vi "Post-Project-Copying Process - Error Handling.vi"(8 "error in":errorcluster, 11 "PluginGenerator_MetaDataObj":refnum<class "PluginGenerator_MetaDataObj.lvclass">) -> (0 "error out":errorcluster, 3 "PluginGenerator_MetaDataObj out":refnum<class "PluginGenerator_MetaDataObj.lvclass">)   [LabVIEW 2023, in "Plugin Generator.lvlib"]
uses:
  Plugin Generator.lvlib
  PluginGenerator_MetaDataObj/PluginGenerator_MetaDataObj.lvclass
  c:/perforce/build/exports/ni/nito/nitoolchainlabview2023eng64/official/export/23.3/23.3.0f52/win/resource/dialog/NewProjectWizard/MetaDataObj/MetaDataObj.lvclass
  <vilib>/Utility/error.llb/DialogType.ctl
  <resource>/dialog/NewProjectWizard/MetaDataObj/MetaDataObj.lvclass/MetaDataObj.ctl
  <resource>/dialog/NewProjectWizard/MetaDataObj/Accessors/Read Project Root.vi
  <resource>/dialog/NewProjectWizard/MetaDataObj/Accessors/Read Project Name.vi
  <vilib>/dlg_ctls.llb/Space Constant.vi
  [Global].vi
  <resource>/dialog/NewProjectWizard/MetaDataObj/Accessors/Read Project Path.vi
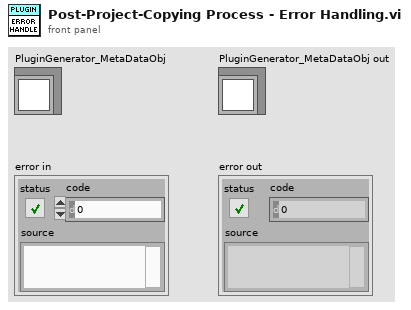
[diagram p1: front panel]
types:
  T1 = typedef "DialogType.ctl" = u16
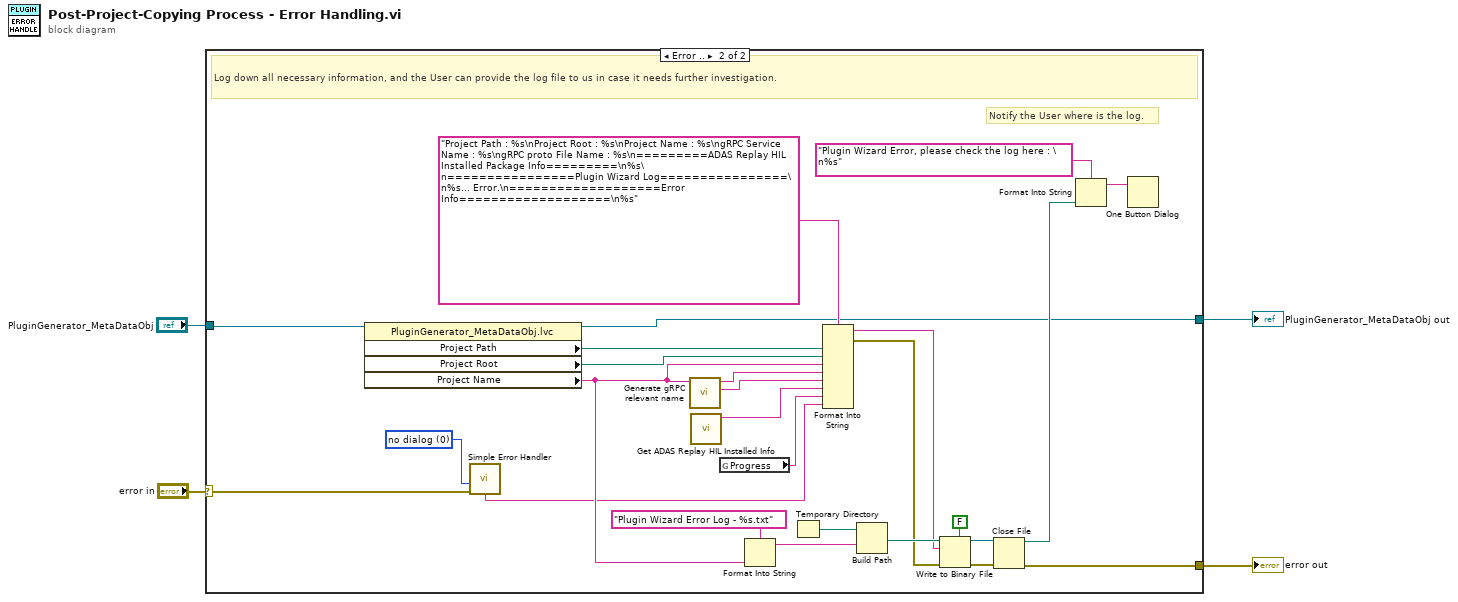
[diagram p0: block diagram]
diagram:
  n1 = case shown="Error .." "error in" {
    selector: "error in" -> [w6 w32]
    tunnel: [w6 w12] -> w4
    tunnel: "PluginGenerator_MetaDataObj" -> [w5 w30]
    tunnel: [w5 w11] -> w1
    frame No Error {
    }
    frame Error {
      w31 = T1 0 items=["no dialog", "OK message", "continue or stop message", "OK message + warnings", "continue/stop + warnings"] ("type of dialog (OK msg:1)")
      # "Notify the User where is the log."
      # "Log down all necessary information, and the User can provide the log file to us in case it needs further investigation."
      n2 = property class="PluginGenerator_MetaDataObj.lvc"(reference=w30) -> (reference out=w11:refnum<class "PluginGenerator_MetaDataObj.lvclass">, "Project Path"=w29:path, "Project Root"=w28:path, "Project Name"=w23:string)  [unwired: 1 in, 1 out]
      n3 = call <vilib>:"Simple Error Handler.vi"("type of dialog (OK msg:1)"=w31, "error in (no error)"=w32) -> ("message"=w9:string)  [unwired: 3 in, 4 out]
      n4 = call "Generate gRPC relevant name.vi"("Project Name"=w23) -> ("gRPC proto File Name"=w26:string, "gRPC Service Name"=w27:string)  [unwired: 9 in]
      n5 = call "Get ADAS Replay HIL Installed Info.vi"() -> ("ADAS Replay HIL pkg info"=w7:string)  [unwired: 11 in]
      n6 = global read "[Global].vi" "Progress"() -> (w8:string)
      n7 = Format Into String(format string="Plugin Wizard Error Log - %s.txt", w23) -> (resulting string=w21:string)  [unwired: 2 in, 1 out]
      n8 = Temporary Directory() -> (w24:path)
      n9 = Format Into String(format string="Project Path : %s\nProject Root : %s\nProject Name : %s\ngRPC Service Name : %s\ngRPC proto File Name : %s\n=========ADAS Replay HIL Installed Package Info=========\n%s\n================Plugin Wizard Log================\n%s... Error.\n===================Error Info===================\n%s", w29, w28, w23, w27, w26, w7, w8, w9) -> (resulting string=w19:string, error out=w18:errorcluster)  [unwired: 2 in]
      n10 = Build Path(base path=w24, name or relative path=w21) -> (appended path=w20:path)
      n11 = Write to Binary File(file (use dialog)=w20, data=w19, error in=w18, 5:FALSE ("prepend array or string size? (T)")) -> (refnum out=w16:refnum<file>, error out=w17:errorcluster)  [unwired: 2 in, 1 out]
      n12 = Close File(refnum=w16, error in=w17) -> (path=w15:path, error out=w12:errorcluster)
      n13 = Format Into String(format string="Plugin Wizard Error, please check the log here : \n%s", w15) -> (resulting string=w13:string)  [unwired: 2 in, 1 out]
      n14 = One Button Dialog(message=w13) -> ()  [unwired: 1 in, 1 out]
    }
  }
  "error out" <- w4
  "PluginGenerator_MetaDataObj out" <- w1
